vi "Flatten.vi"(8 "error in (no error)":errorcluster, 11 "Dummy Scan in":refnum<class "Dummy Scan.lvclass">) -> (0 "error out":errorcluster, 3 "Dummy Scan out":refnum<class "Dummy Scan.lvclass">)   [LabVIEW 2017, in "Dummy Scan.lvclass"]
uses:
  Dummy Scan.lvclass
  Dummy Scan.lvclass/Dummy Scan.ctl
  Global/File Locations.vi
  Scanner/Scanner.lvclass
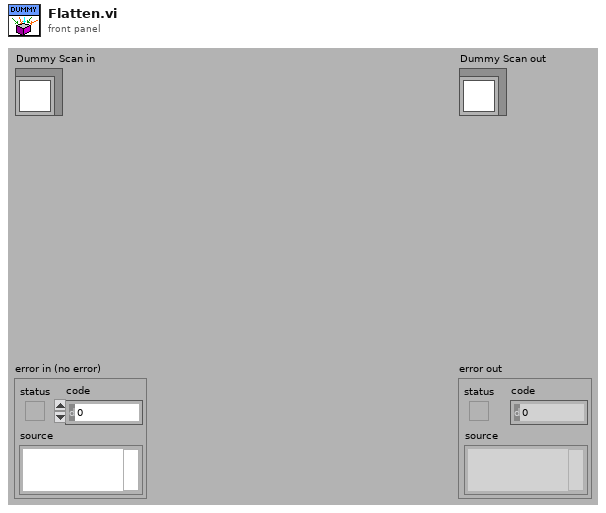
[diagram p1: front panel]
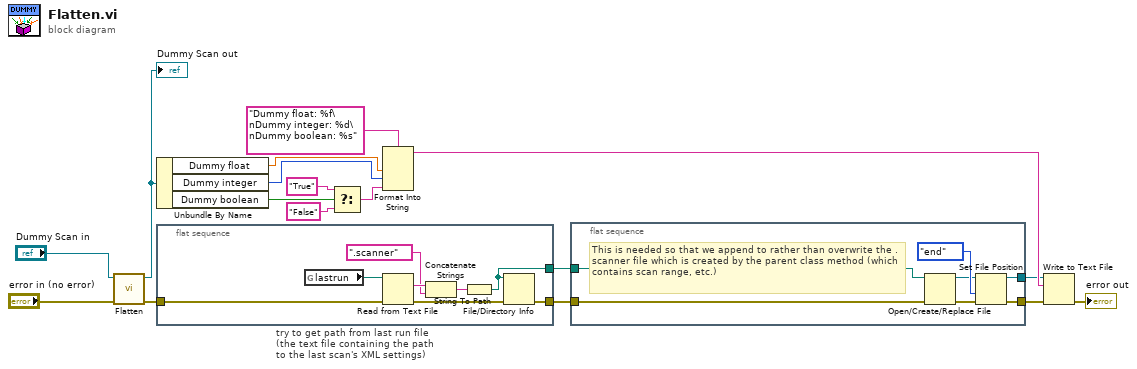
[diagram p0: block diagram]
diagram:
  n1 = call-parent "Flatten.vi"("error in (no error)"="error in (no error)", "Scanner in"="Dummy Scan in") -> ("error out"=w15:errorcluster, "Scanner out"=w13:refnum<class "Dummy Scan.lvclass">)  [unwired: 8 in]
  "Dummy Scan out" <- w13
  n2 = Unbundle By Name(w13) -> ("Dummy float"=w10:dbl, "Dummy integer"=w2:i16, "Dummy boolean"=w5:bool)
  n3 = flat-sequence "try to get path from last run file\n(the text file containing the path\nto the last scan's XML settings)" {
    tunnel: [w25] -> w7
    tunnel: [w22] -> w6
    tunnel: w15 -> [w21]
    frame #0 {
      n4 = global read "File Locations.vi" "lastrun"() -> (w24:path)
      n5 = Read from Text File(file (use dialog)=w24, error in=w21) -> (text=w20:string, error out=w23:errorcluster)  [unwired: 4 out]
      n6 = Concatenate Strings(w20, ".scanner") -> (w18:string)
      n7 = String To Path(string=w18) -> (path=w25:path)
      n8 = File/Directory Info(path=w25, error in=w23) -> (error out=w22:errorcluster)  [unwired: 6 out]
    }
  }
  n9 = Select(t="True", s=w5, f="False") -> (s? t:f=w1:string)
  n10 = Format Into String(format string="Dummy float: %f\nDummy integer: %d\nDummy boolean: %s", w10, w2, w1) -> (resulting string=w11:string)  [unwired: 2 in, 1 out]
  n11 = flat-sequence {
    tunnel: [w31] -> w9
    tunnel: [w30] -> w8
    tunnel: w7 -> [w29]
    tunnel: w6 -> [w28]
    frame #0 {
      # "This is needed so that we append to rather than overwrite the .scanner file which is created by the parent class method (which contains scan range, etc.)"
      n12 = Open/Create/Replace File(file path (use dialog)=w29, error in=w28) -> (refnum out=w27:refnum<file>, error out=w26:errorcluster)  [unwired: 4 in, 1 out]
      n13 = Set File Position(refnum=w27, from (0:start)=enum16{"start", "end", "current"}."end", error in=w26) -> (refnum out=w30:refnum<file>, error out=w31:errorcluster)  [unwired: 1 in]
    }
  }
  n14 = Write to Text File(file (use dialog)=w8, text=w11, error in=w9) -> (error out=→"error out":errorcluster)  [unwired: 1 in, 2 out]
